vi "Dequeue Master and Local.vi"(8 "error in (no error)":errorcluster, 10 "Master":refnum<queue>, 11 "UI In":refnum<queue>) -> (0 "error out":errorcluster, 1 "Message Data":variant, 2 "Message":string, 3 "UI Out":refnum<queue>)   [LabVIEW 2013, in "Yokogawa.lvlib" / "YKPZ400 Message Queue.lvlib"]
uses:
  YKPZ400 Message Queue.lvlib
  Message Cluster.ctl
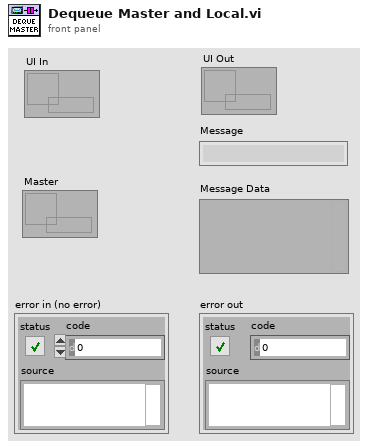
[diagram p1: front panel]
types:
  T1 = typedef "Yokogawa.lvlib/YKPZ400 Message Queue.lvlib/Message Cluster.ctl" = cluster{"Message":string, "Message Data":variant}
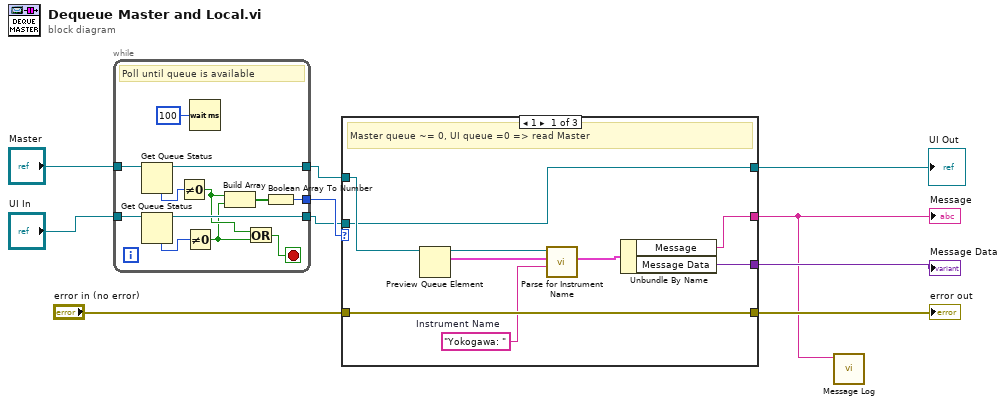
[diagram p0: block diagram]
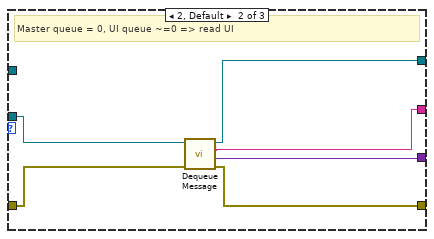
[diagram p2: hidden frame]
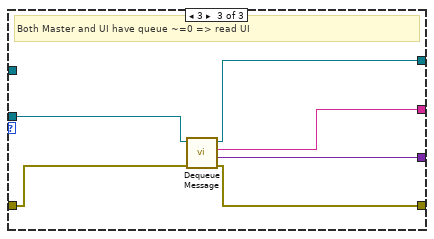
[diagram p3: hidden frame]
diagram:
  n1 = while {
    tunnel: "UI In" -> [w22]
    tunnel: "Master" -> [w19]
    tunnel: [w17] -> w10
    tunnel: [w16] -> w9
    tunnel: [w15] -> w8
    stop <- w13 stop-if-true
    # "Poll until queue is available"
    n2 = Get Queue Status(queue=w19) -> (queue out=w16:refnum<queue>, # elements in queue=w20:i32)  [unwired: 2 in, 6 out]
    n3 = Get Queue Status(queue=w22) -> (queue out=w15:refnum<queue>, # elements in queue=w21:i32)  [unwired: 2 in, 6 out]
    n4 = Not Equal To 0?(x=w20) -> (x != 0?=w12:bool)
    n5 = Not Equal To 0?(x=w21) -> (x != 0?=w11:bool)
    n6 = Wait (ms)(milliseconds to wait=u32 100) -> ()  [unwired: 1 out]
    n7 = Build Array(w12, w11) -> (w18:bool[])
    n8 = Or(x=w12, y=w11) -> (x .or. y?=w13:bool)
    n9 = Boolean Array To Number(Boolean array=w18) -> (number=w17:u32)
  }
  n10 = case shown="1" w10 {
    tunnel: w9 -> [w28 _ _]
    tunnel: w8 -> [w27 w37 w43]
    tunnel: "error in (no error)" -> [w29 w36 w42]
    tunnel: [w27 w32 w38] -> w4
    tunnel: [w31 w33 w39] -> w1
    tunnel: [w30 w34 w40] -> w5
    tunnel: [w29 w35 w41] -> w6
    frame 1 {
      w23 = "Yokogawa: "  # Instrument Name
      # "Master queue ~= 0, UI queue =0 => read Master"
      n11 = Preview Queue Element(queue=w28) -> (queue out=w25:refnum<queue>, element=w24:T1)  [unwired: 2 in, 2 out]
      n12 = call "Parse for Instrument Name.vi"("Instrument Name"=w23, "Message In"=w24, "UI"=w25) -> ("Message Out"=w26:T1)  [unwired: 8 in]
      n13 = Unbundle By Name(w26) -> ("Message"=w31:string, "Message Data"=w30:variant)
    }
    frame 2, Default {
      # "Master queue = 0, UI queue ~=0 => read UI"
      n14 = call "Dequeue Message.vi"("error in (no error)"=w36, "Message Queue"=w37) -> ("error out"=w35:errorcluster, "Message Data"=w34:variant, "Message"=w33:string, "dup Message Queue"=w32:refnum<queue>)  [unwired: 6 in]
    }
    frame 3 {
      # "Both Master and UI have queue ~=0 => read UI"
      n15 = call "Dequeue Message.vi"("error in (no error)"=w42, "Message Queue"=w43) -> ("error out"=w41:errorcluster, "Message Data"=w40:variant, "Message"=w39:string, "dup Message Queue"=w38:refnum<queue>)  [unwired: 6 in]
    }
  }
  "error out" <- w6
  "Message" <- w1
  "Message Data" <- w5
  "UI Out" <- w4
  n16 = call "Message Log.vi"("Message"=w1) -> ()  [unwired: 11 in]
